vi "XML_fast.vi"(5 "HV Cluster":T2={"HV Power On/Off"=[FALSE, FALSE, FALSE, FALSE, FALSE, FALSE, FALSE, FALSE], "Set Voltage"=["0", "0", "0", "0", "0", "0", "0", "0"], "HV Tolerance (%)"=1.0, "Current"=[]}, 6 "Channel Cluster":T1={"det_type"=["", "", "", "", "", "", "", ""], "Serial numbers"=["", "", "", "", "", "", "", ""], "Sources"=["", "", "", "", "", "", "", ""], "Trigger level"=[4000, 4000, 4000, 4000, 4000, 4000, 4000, 4000], "Data Record On/Off"=[FALSE, FALSE, FALSE, FALSE, FALSE, FALSE, FALSE, FALSE, FALSE, FALSE, FALSE, FALSE, FALSE, FALSE, FALSE, FALSE], "Number of Channels"=8}, 7 "DAQ Info Cluster":T3={"Data Chunks per File"=1000, "Samples per Waveform"=95, "Pretrigger Samples"=15, "circular buffer length (samples)"=1000, "Waveforms per Data Chunk"=5000} {"Waveforms per Data Chunk" format="%.2p"}, 8 "Testpulse Cluster":T4={"Master Pulser On/Off"=FALSE, "Testpulse Turnaround Time (samples)"=14, "Pulse Separation (samples)"=0, "Pulse duration (samples)"=0}, 9 "IP Address of NIST Time Server":string(combo), 10 "NIST Time":u64, 11 "General Cluster":cluster{"Location":i16} {"Location" items=["Purdue", "NIKHEF", "Zurich", "???"]}) -> (2 "XML String":string)   [LabVIEW 2012]
uses:
  hv cluster control.ctl
panel:
  # "Channel 0"
  # "Channel 1"
  # "Channel 2"
  # "Channel 3"
  # "Channel 4"
  # "Channel 5"
  # "Channel 6"
  # "Channel 7"
  # "Waveform/Data Chunk information"
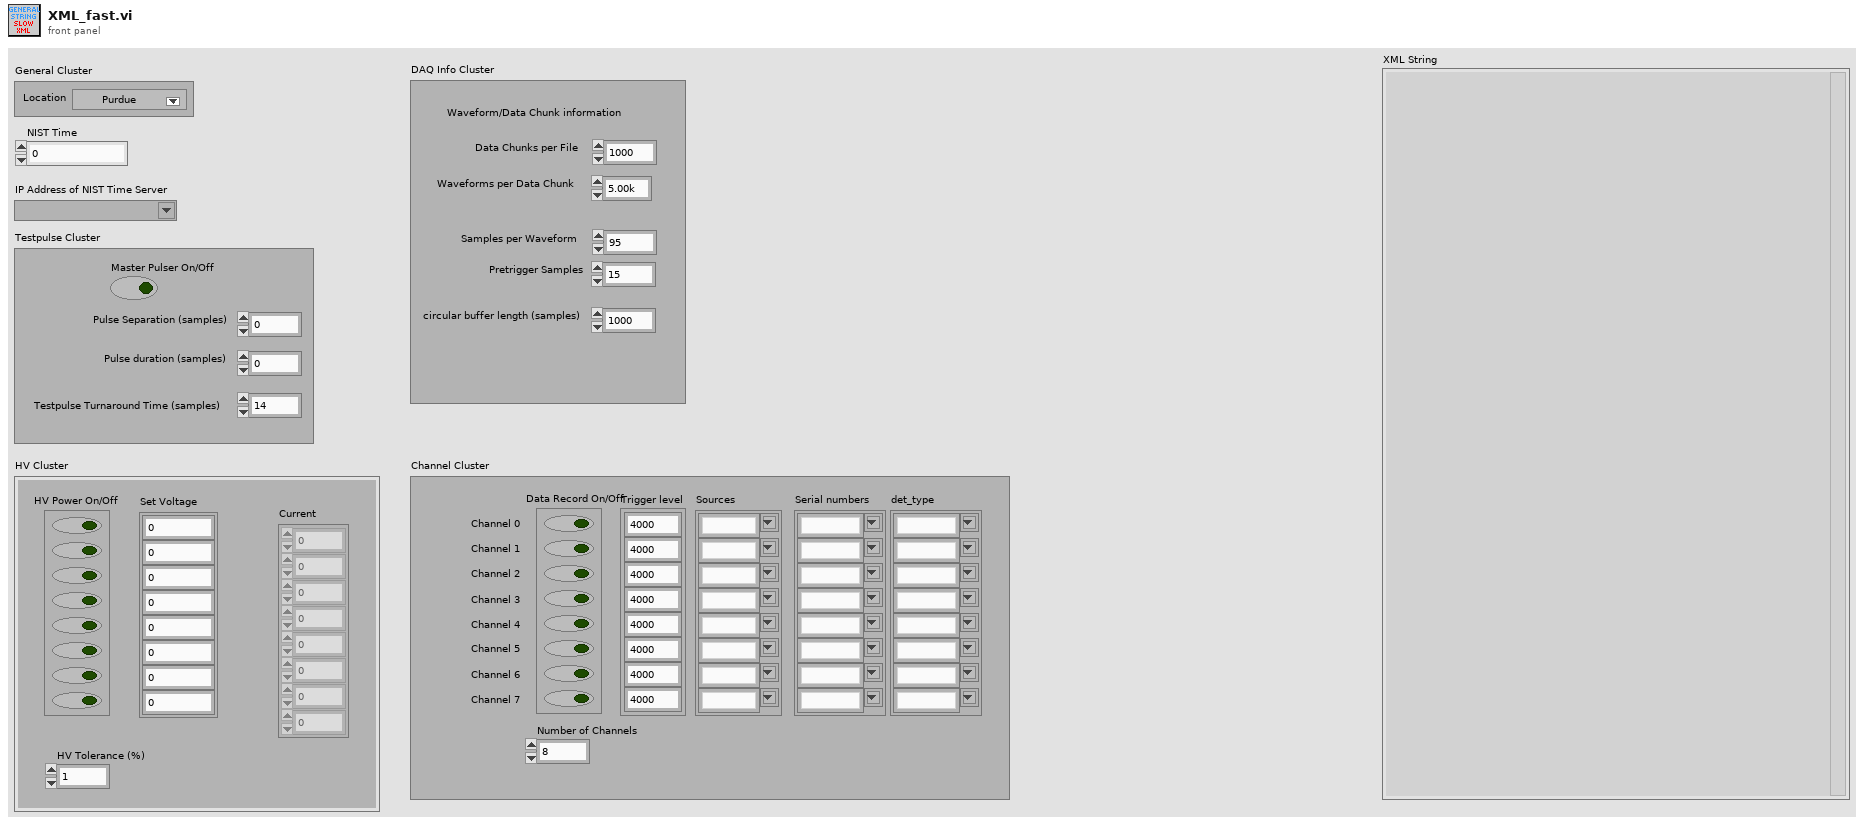
[diagram p1: front panel]
types:
  T1 = cluster{"det_type":string[], "Serial numbers":string[], "Sources":string[], "Trigger level":i16[], "Data Record On/Off":bool[], "Number of Channels":u8}
  T2 = typedef "hv cluster control.ctl" = cluster{"HV Power On/Off":bool[], "Set Voltage":string[], "HV Tolerance (%)":dbl, "Current":dbl[]}
  T3 = cluster{"Data Chunks per File":u32, "Samples per Waveform":u32, "Pretrigger Samples":u32, "circular buffer length (samples)":u32, "Waveforms per Data Chunk":u32}
  T4 = cluster{"Master Pulser On/Off":bool, "Testpulse Turnaround Time (samples)":u32, "Pulse Separation (samples)":u32, "Pulse duration (samples)":u32}
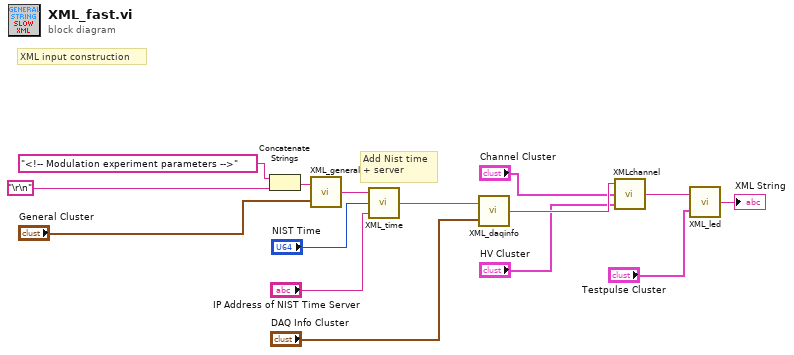
[diagram p0: block diagram]
diagram:
  # "Add Nist time\n+ server"
  # "XML input construction"
  n1 = Concatenate Strings("<!-- Modulation experiment parameters -->", "\r\n") -> (w9:string)
  n2 = call "XML_general.vi"("General Cluster"="General Cluster", "Input String"=w9) -> ("Output String"=w8:string)
  n3 = call "XML_time.vi"("IP Address of NIST Time Server"="IP Address of NIST Time Server", "NIST Time"="NIST Time", "Input String"=w8) -> ("Output String"=w7:string)
  n4 = call "XML_daqinfo.vi"("DAQ Info Cluster"="DAQ Info Cluster", "Input String"=w7) -> ("Output String"=w6:string)
  n5 = call "XMLchannel.vi"("HV Cluster"="HV Cluster", "Channel Cluster"="Channel Cluster", "Previous XML string"=w6) -> ("Output String"=w12:string)
  n6 = call "XML_led.vi"("Testpulse Cluster"="Testpulse Cluster", "Input String"=w12) -> ("Output String"=→"XML String":string)
